vi "ShiftGlobals.vi"() -> ()   [LabVIEW 2015]
panel:
  out "DriveSpeed":dbl
  out "HoldLowGear":bool
  out "HighGear":bool
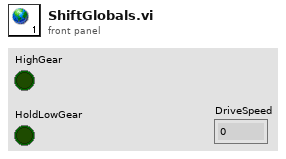
[diagram p1: front panel]
diagram:
